vi "launch_console.vi"(8 "error (in)":errorcluster, 11 "console.provider.lvclass":refnum<class "console.provider.lvclass">) -> (0 "error (out)":errorcluster, 3 "console.provider (out)":refnum<class "console.provider.lvclass">)   [LabVIEW 2021, in "console.provider.lvclass"]
uses:
  console.provider.lvclass
  Z:/Projects/PCCS/labview-system-logging/source/system.logging.provider/system.logging.provider.lvclass
  system.logging.provider.lvclass/system.logging.provider.ctl
  console.provider.lvclass/console.provider.ctl
  system.logging.provider.lvclass
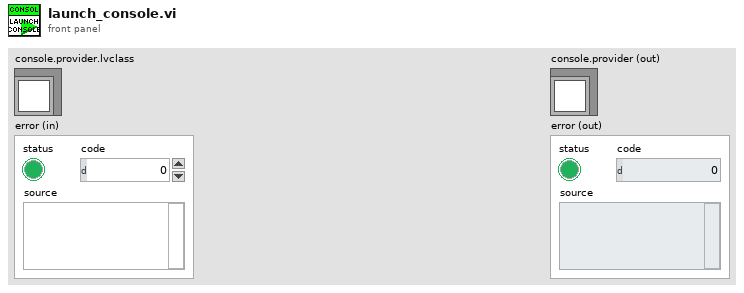
[diagram p1: front panel]
types:
  T1 = typedef "system.logging.lvclass/severity.ctl" = enum8{"trace", "debug", "info", "warning", "error"}
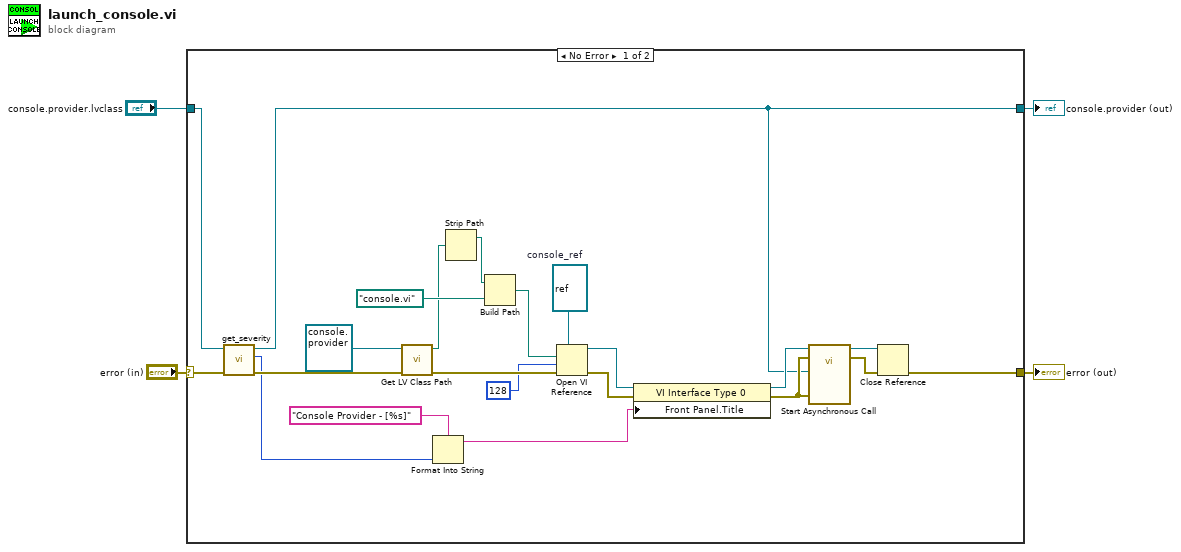
[diagram p0: block diagram]
diagram:
  n1 = case shown="No Error" "error (in)" {
    selector: "error (in)" -> [w11 w28]
    tunnel: [w22 w28] -> w1
    tunnel: [w9 w27] -> w3
    tunnel: "console.provider.lvclass" -> [w10 w27]
    frame No Error {
      w18 = refnum<vi> refnum  # console_ref
      n2 = call "get_severity.vi"("error in (no error)"=w11, "system.logging.provider in"=w10) -> ("error out"=w8:errorcluster, "severity"=w6:T1, "system.logging.provider out"=w9:refnum<class "console.provider.lvclass">)  [unwired: 7 in]
      n3 = call <vilib>:"Get LV Class Path.vi"("error in (no error)"=w8, "object"=refnum<class "console.provider.lvclass"> refnum ("console.provider.lvclass")) -> ("error out"=w25:errorcluster, "class path"=w21:path)  [unwired: 8 in]
      n4 = Format Into String(format string="Console Provider - [%s]" ("Front Panel Window:Title"), w6) -> (resulting string=w5:string)  [unwired: 2 in, 1 out]
      n5 = Strip Path(path=w21) -> (stripped path=w20:path)  [unwired: 1 out]
      n6 = Build Path(base path=w20, name or relative path=path "console.vi") -> (appended path=w23:path)
      n7 = Open VI Reference(type specifier VI Refnum (for type only)=w18, vi path=w23, options=128, error in (no error)=w25) -> (vi reference=w15:refnum<vi>, error out=w13:errorcluster)  [unwired: 2 in]
      n8 = property class="VI Interface Type 0"(reference=w15, error in=w13, "Front Panel.Title"=w5) -> (reference out=w14:refnum<vi>, error out=w12:errorcluster)
      n9 = call-by-ref "Start Asynchronous Call"(reference=w14, error in=w12, 8:"error in (no error)"=w12, "console.provider in"=w9) -> (reference out=w17:refnum<vi>, error out=w16:errorcluster)  [unwired: 9 in, 1 out]
      n10 = Close Reference(reference=w17, error in (no error)=w16) -> (error out=w22:errorcluster)
    }
    frame Error {
    }
  }
  "console.provider (out)" <- w3
  "error (out)" <- w1
